vi "DivisionVI.vi"() -> ()   [LabVIEW 2019]
panel:
  out "Result":dbl
  out "Remainder":dbl
  out "Result":dbl
  in  "y":dbl
  in  "x":dbl
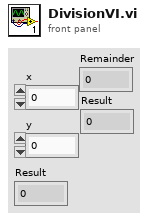
[diagram p1: front panel]
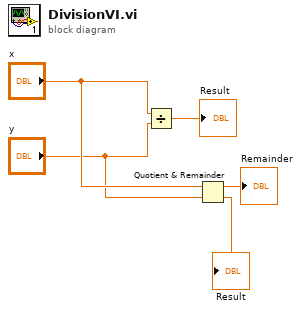
[diagram p0: block diagram]
diagram:
  n1 = Divide(x="x", y="y") -> (x/y=→"Result":dbl)
  n2 = Quotient & Remainder(x="x", y="y") -> (x-y*floor(x/y)=→"Remainder":dbl, floor(x/y)=→"Result":dbl)
